vi "sort names.vi"(8 "error in":errorcluster, 9 "Name":string) -> (0 "error out":errorcluster, 1 "display value?":bool)   [LabVIEW 2016, in "flat top.lvlib"]
doc: "This vi sorts through the names of a vis' control and only displays the ones that are used for flat topping"
uses:
  flat top.lvlib
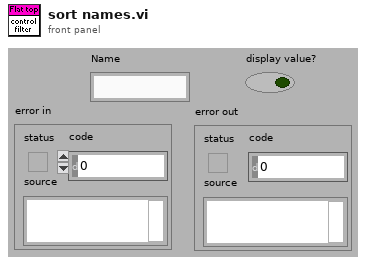
[diagram p1: front panel]
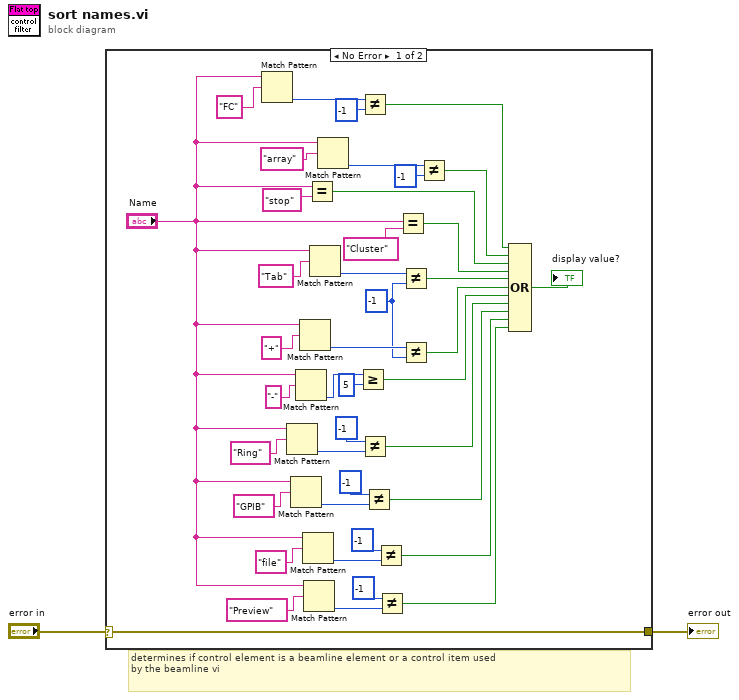
[diagram p0: block diagram]
diagram:
  # "determines if control element is a beamline element or a control item used\nby the beamline vi"
  n1 = case shown="No Error" "error in" {
    selector: "error in" -> [w25 w45]
    tunnel: [w25 w45] -> w1
    frame No Error {
      w30 = -1 ("y")
      n2 = Match Pattern(string="Name", regular expression="FC") -> (offset past match=w39:i32)  [unwired: 4 out]
      n3 = Match Pattern(string="Name", regular expression="Ring") -> (offset past match=w33:i32)  [unwired: 4 out]
      n4 = Match Pattern(string="Name", regular expression="GPIB") -> (offset past match=w14:i32)  [unwired: 4 out]
      n5 = Match Pattern(string="Name", regular expression="-") -> (offset past match=w44:i32)  [unwired: 4 out]
      n6 = Match Pattern(string="Name", regular expression="+") -> (offset past match=w31:i32)  [unwired: 4 out]
      n7 = Match Pattern(string="Name", regular expression="file") -> (offset past match=w11:i32)  [unwired: 4 out]
      n8 = Match Pattern(string="Name", regular expression="Preview") -> (offset past match=w6:i32)  [unwired: 4 out]
      n9 = Equal?(x="Name", y="stop") -> (x = y?=w21:bool)
      n10 = Match Pattern(string="Name", regular expression="Tab") -> (offset past match=w41:i32)  [unwired: 4 out]
      n11 = Match Pattern(string="Name", regular expression="array") -> (offset past match=w26:i32)  [unwired: 4 out]
      n12 = Greater Or Equal?(x=w44, y=5) -> (x >= y?=w17:bool)
      n13 = Not Equal?(x=w39, y=-1) -> (x != y?=w23:bool)
      n14 = Not Equal?(x=-1 ("y"), y=w33) -> (x != y?=w16:bool)
      n15 = Not Equal?(x=-1 ("y"), y=w14) -> (x != y?=w9:bool)
      n16 = Not Equal?(x=-1 ("y"), y=w11) -> (x != y?=w8:bool)
      n17 = Not Equal?(x=-1 ("y"), y=w6) -> (x != y?=w3:bool)
      n18 = Equal?(x="Name", y="Cluster" ("regular expression")) -> (x = y?=w20:bool)
      n19 = Not Equal?(x=w41, y=w30) -> (x != y?=w19:bool)
      n20 = Not Equal?(x=w31, y=w30) -> (x != y?=w18:bool)
      n21 = Not Equal?(x=w26, y=-1) -> (x != y?=w22:bool)
      n22 = Compound Arithmetic op=OR(w23, w22, w21, w20, w19, w18, w17, w16, w9, w8, w3) -> (→"display value?":bool)
    }
    frame Error {
    }
  }
  "error out" <- w1
